vi "loop_while.vi"(4 "Stop_program":bool, 5 "error in (no error)":errorcluster, 6 "P_max":dbl, 7 "Number of samples":i32, 8 "V_max":dbl, 9 "V_min":dbl) -> (0 "error out":errorcluster, 1 "progress":u8(slide) scale=0.0..100.0, 2 "Current":dbl[](array[numeric]), 3 "Voltage":dbl[](array[numeric]))   [LabVIEW 2020]
uses:
  <vilib>/Analysis/NI_AALBase.lvlib
  <vilib>/Analysis/1siggen.llb/Ramp Pattern by Samples.vi
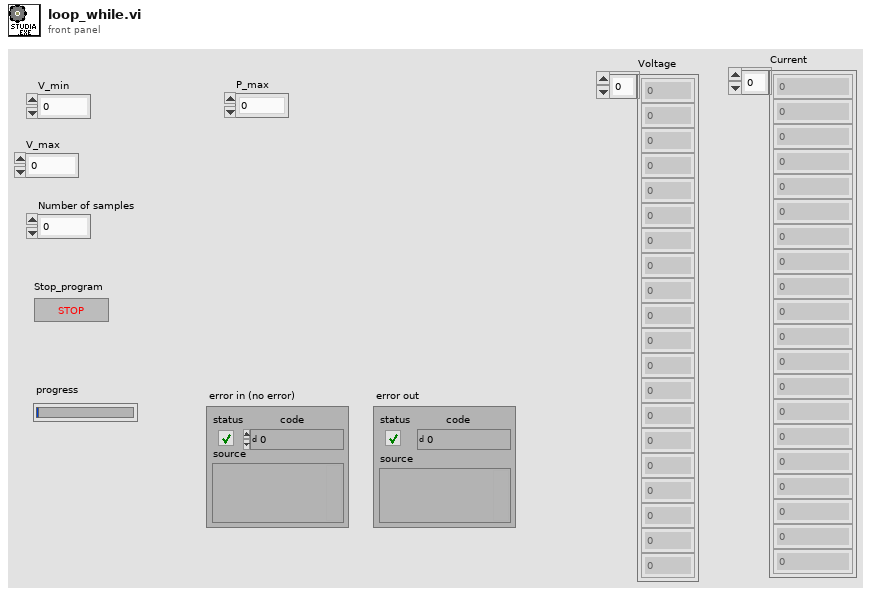
[diagram p1: front panel]
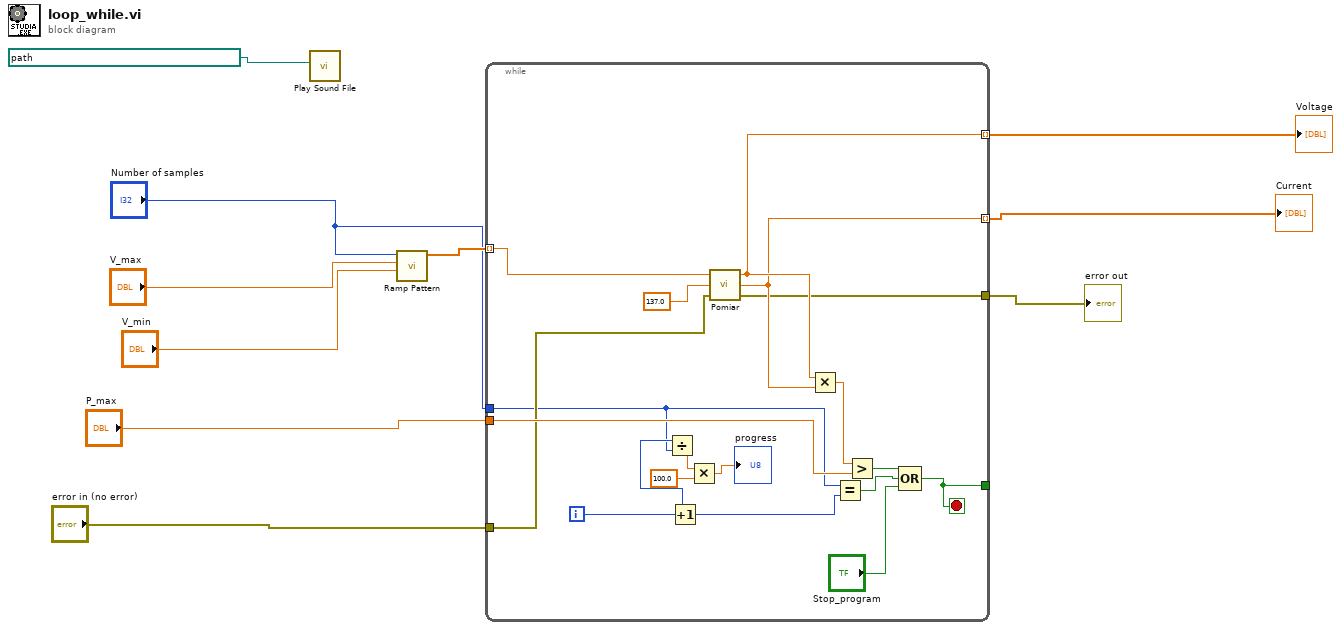
[diagram p0: block diagram]
diagram:
  n1 = call <vilib>:"Play Sound File.vi"("path"=path "C:/Users/Kopeć/Desktop/SAiPT/long.wav" ("Path")) -> ()  [unwired: 9 in, 2 out]
  n2 = call-poly <vilib>:"Ramp Pattern.vi"("start"="V_min", "end"="V_max", "samples"="Number of samples") -> ("Ramp Pattern"=w8:dbl[])  [unwired: 7 in, 1 out]
  n3 = while {
    tunnel: w8 -> [w28] mode=indexing
    tunnel: "P_max" -> [w26]
    tunnel: [w25] -> w6 mode=indexing
    tunnel: [w24] -> w5 mode=indexing
    tunnel: "Number of samples" -> [w15]
    tunnel: [w19] -> w3
    tunnel: "error in (no error)" -> [w18]
    tunnel: [w17] -> _
    i -> [w22]
    stop <- w17 stop-if-true
    n4 = Increment(x=w22) -> (x+1=w16:i32)
    n5 = Divide(x=w16, y=w15) -> (x/y=w14:dbl)
    n6 = Multiply(x=w14, y=100.0) -> (x*y=→"progress":dbl)
    n7 = call "Pomiar.vi"("error in (no error)"=w18, "Resistance"=137.0, "Voltage"=w28) -> ("error out"=w19:errorcluster, "Current output"=w24:dbl, "Voltage output"=w25:dbl)
    n8 = Multiply(x=w25, y=w24) -> (x*y=w27:dbl)
    n9 = Equal?(x=w15, y=w16) -> (x = y?=w20:bool)
    n10 = Greater?(x=w27, y=w26) -> (0:w21:bool)
    n11 = Compound Arithmetic op=OR(w21, w20, "Stop_program") -> (w17:bool)
  }
  "Voltage" <- w6
  "Current" <- w5
  "error out" <- w3
